vi "heatmap_from_raw.vi"() -> ()   [LabVIEW 2015]
uses:
  <vilib>/Utility/file.llb/Read Delimited Spreadsheet (DBL).vi
panel:
  out "Intensity Graph 2":dbl[][](graph)
  out "size(s)":i64[](array[numeric])
  out "all rows":dbl[][](array[numeric])
  in  "Path":path=path "C:/Users/arnold/Documents/labview/afm_imaging/grating01.csv"
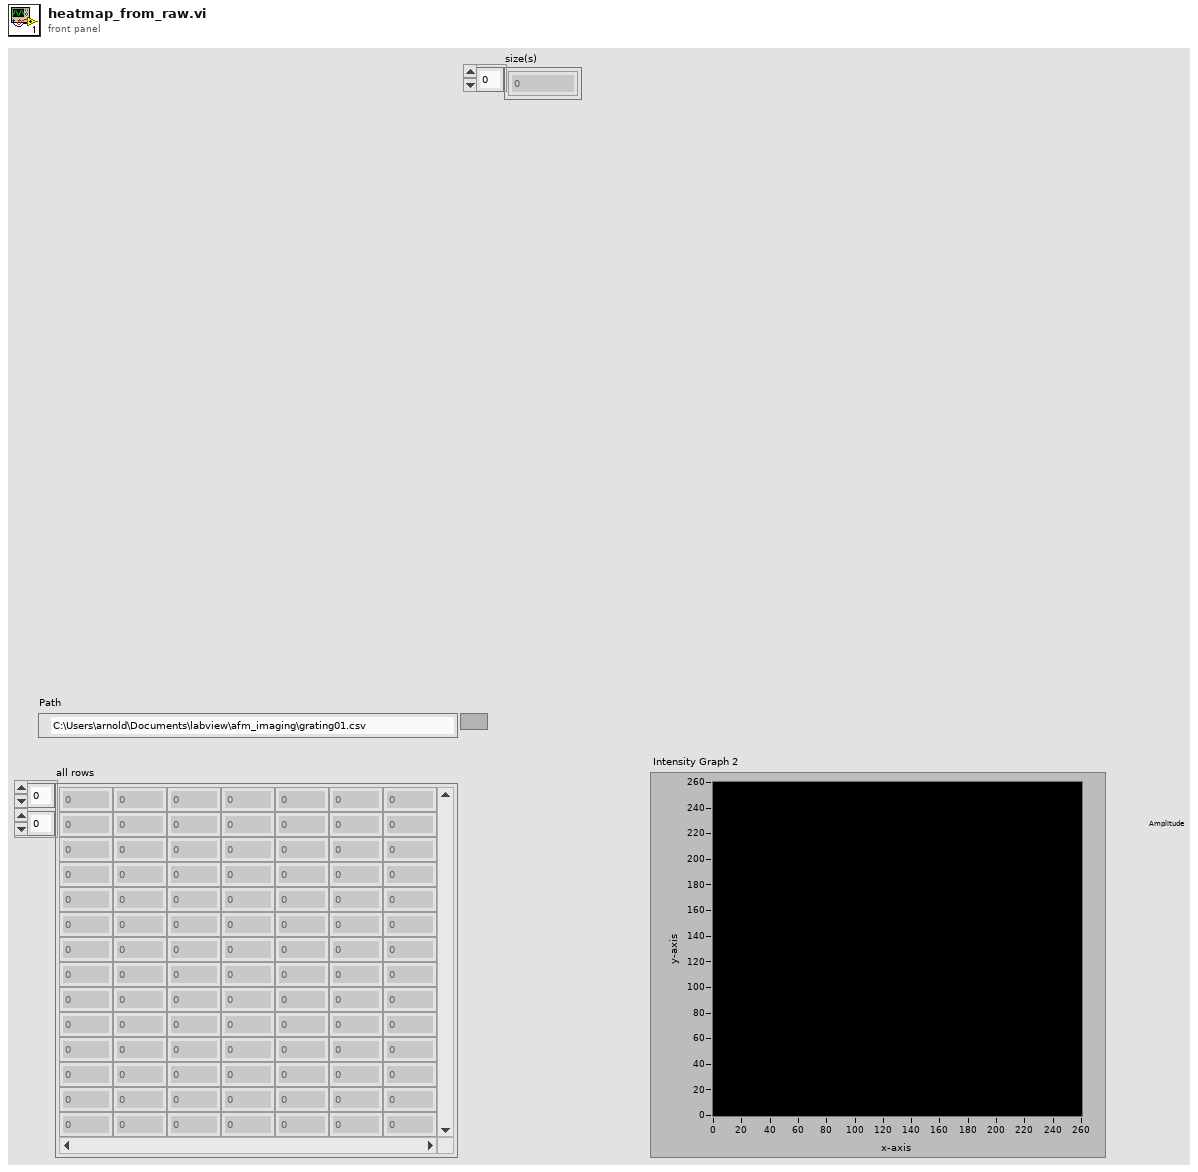
[diagram p1: front panel]
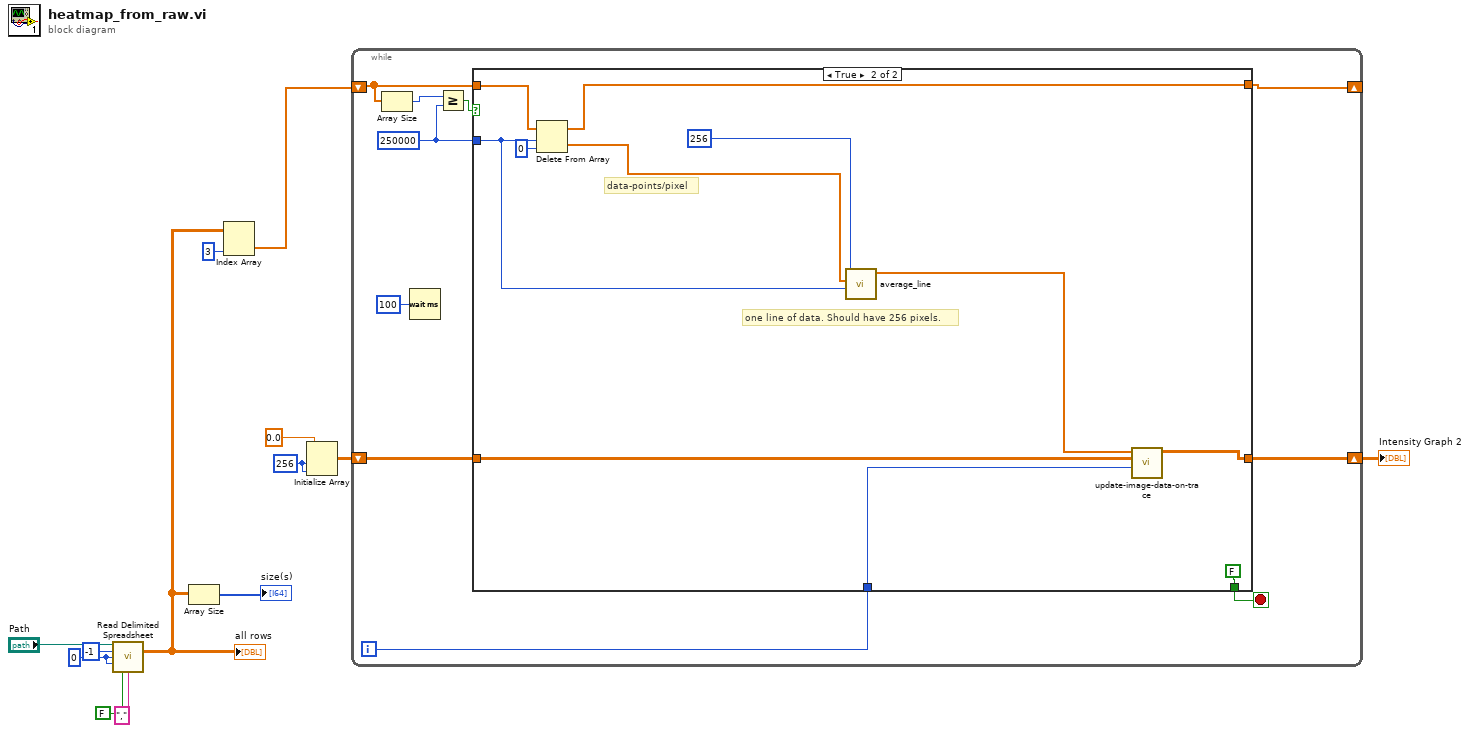
[diagram p0: block diagram]
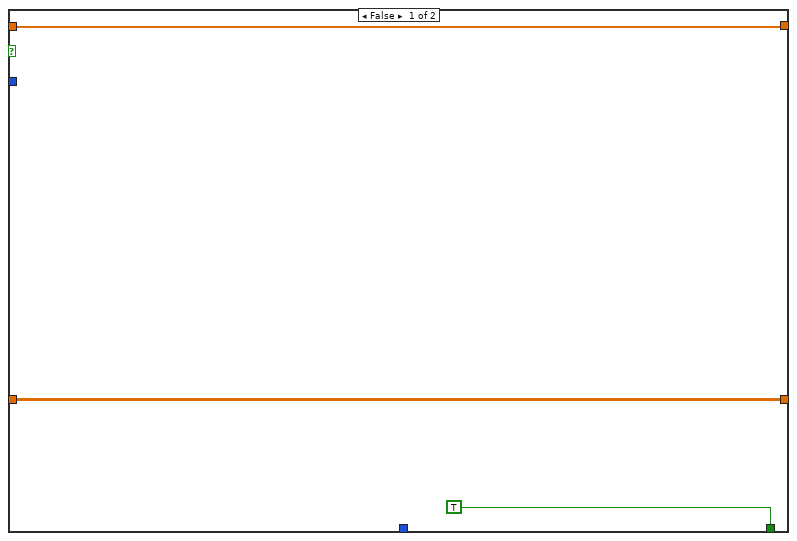
[diagram p2: hidden frame]
diagram:
  w4 = 256 ("dimension size")
  w10 = 0 ("start of read offset (chars.:0)")
  n1 = call-poly <vilib>:"Read Delimited Spreadsheet.vi"("file path (dialog if empty)"="Path", "number of rows (all:-1)"=-1, "start of read offset (chars.:0)"=w10, "max characters/row  (no limit:0)"=w10, "transpose? (F)"=FALSE, "delimiter (\\t)"="," ("delimiter (\\t)")) -> ("all rows"=w7:dbl[][])  [unwired: 4 in, 5 out]
  "all rows" <- w7
  n2 = Array Size(array=w7) -> (size(s)=→"size(s)":i32[])
  n3 = Index Array(array=w7, index (col)=3 ("disabled index (col)")) -> (element=w5:dbl[])  [unwired: 1 in]
  n4 = Initialize Array(0.0 ("element"), w4, w4) -> (w2:dbl[][])
  n5 = while {
    shift-right: [w23] -> _
    shift-left: w5 -> [w22]
    shift-right: [w16] -> w1
    shift-left: w2 -> [w17]
    i -> [w14]
    stop <- w18 stop-if-true
    w20 = 250000 ("points_per_line")
    n6 = Array Size(array=w22) -> (size(s)=w21:i32)
    n7 = Wait (ms)(milliseconds to wait=u32 100) -> ()  [unwired: 1 out]
    n8 = Greater Or Equal?(x=w21, y=w20) -> (x >= y?=w19:bool)
    n9 = case shown="True" w19 {
      tunnel: [w24 w36] -> w23
      tunnel: w22 -> [w24 w35]
      tunnel: w20 -> [_ w27]
      tunnel: [TRUE FALSE] -> w18
      tunnel: w17 -> [w25 w30]
      tunnel: [w25 w31] -> w16
      tunnel: w14 -> [_ w28]
      frame False {
      }
      frame True {
        # "data-points/pixel"
        # "one line of data. Should have 256 pixels."
        n10 = Delete From Array(array=w35, length=w27, index=0) -> (deleted portion=w33:dbl[], array with subset deleted=w36:dbl[])
        n11 = call "average_line.vi"("data-pts-per-line"=w27, "raw-data-row"=w33, "number-of-pixels"=256 ("points_per_line")) -> ("avg-data-row"=w29:dbl[])  [unwired: 8 in]
        n12 = call "update-image-data-on-trace.vi"("iterator"=w28, "master-image-data-n"=w30, "avg-data-row"=w29) -> ("master-image-data-out"=w31:dbl[][])  [unwired: 8 in]
      }
    }
  }
  "Intensity Graph 2" <- w1
